vi "Grouped Channel History (LV Dbl).vi"(4 "End":dbl, 6 "Start":dbl, 10 "Grouped Channels":map{string, string[]}(c390), 11 "Historian Module in":refnum<class "Historian Module.lvclass">) -> (2 "Local History":T1, 3 "Historian Module out":refnum<class "Historian Module.lvclass">)   [LabVIEW 2020, in "VolatusHistorian.lvlib" / "Historian Module.lvclass"]
uses:
  Historian Module.lvclass
  Historian Module.lvclass/Historian Module.ctl
  Channel History (LV Dbl).ctl
  VolatusHistorian.lvlib
  History Data (LV Dbl).ctl
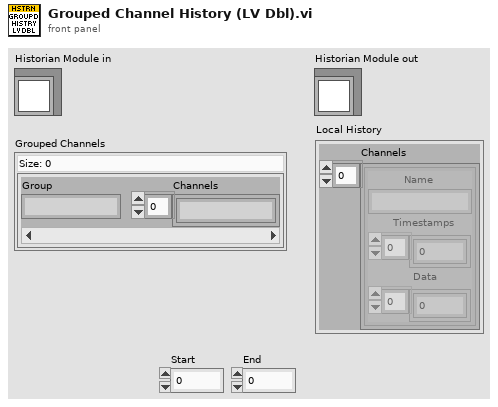
[diagram p1: front panel]
types:
  T1 = typedef "VolatusHistorian.lvlib/History Data (LV Dbl).ctl" = cluster{"Channels":T2[]}
  T2 = typedef "VolatusHistorian.lvlib/Channel History (LV Dbl).ctl" = cluster{"Name":string, "Timestamps":dbl[], "Data":dbl[]}
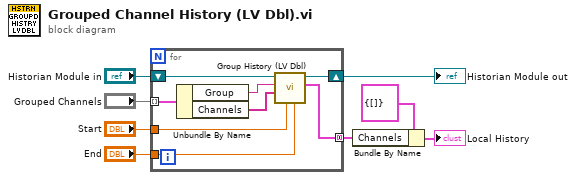
[diagram p0: block diagram]
diagram:
  n1 = for {
    tunnel: "Grouped Channels" -> [w15] mode=indexing
    tunnel: "Start" -> [w11]
    tunnel: "End" -> [w10]
    shift-right: [w14] -> w4
    shift-left: "Historian Module in" -> [w16]
    tunnel: [w9] -> w1 mode=concatenating
    n2 = Unbundle By Name(w15) -> ("Group"=w13:string, "Channels"=w12:string[])
    n3 = call "Group History (LV Dbl).vi"("End"=w10, "Start"=w11, "Channels"=w12, "Group"=w13, "Historian Module in"=w16) -> ("Data"=w9:T2[], "Historian Module out"=w14:refnum<class "Historian Module.lvclass">)  [unwired: 5 in]
  }
  "Historian Module out" <- w4
  n4 = Bundle By Name(cluster=T1 {"Channels"=[]} ("Local History"), "Channels"=w1) -> (→"Local History":T1)
